vi "File_ToClass.vi"(8 "error in (no error)":errorcluster, 11 "Item Ref in":T1 format="%.0x") -> (0 "error out":errorcluster, 2 "Channels":T1[](array[typedef]) format="%.0x", 3 "File out":refnum<class "File.lvclass">)   [LabVIEW 2024, in "Embedded TDMS Logger System Explorer.lvlib"]
doc: "Creates a file class from the VeriStand System Definition File Custom Device defined by the item ref in."
uses:
  Embedded TDMS Logger System Explorer.lvlib
  <vilib>/NI VeriStand/Custom Device API/Custom Device Item Ref.ctl
  Shared/File Classes/File/File.lvclass
  Shared/File Classes/Meta Data.ctl
  <vilib>/NI VeriStand/Custom Device API/Get Item Property (String).vi
  <vilib>/NI VeriStand/Custom Device API/Get Item Property (Variant).vi
  Shared/Constants.vi
  Shared/File Classes/Group/Group.lvclass
  <vilib>/NI VeriStand/Custom Device API/Custom Device API.lvlib
  Shared/Embedded TDMS Logger Shared.lvlib
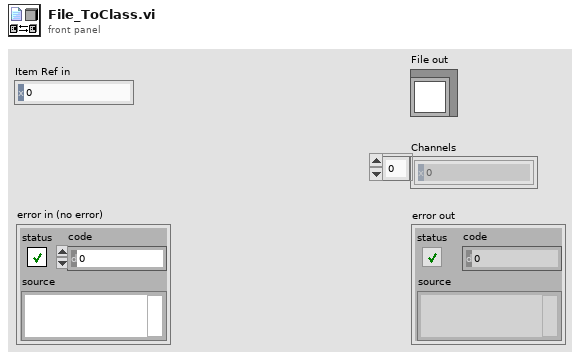
[diagram p1: front panel]
types:
  T1 = typedef "Custom Device API.lvlib/Custom Device Item Ref.ctl" = u64
  T2 = typedef "Meta Data.ctl" = cluster{"Key":string, "Value":string}
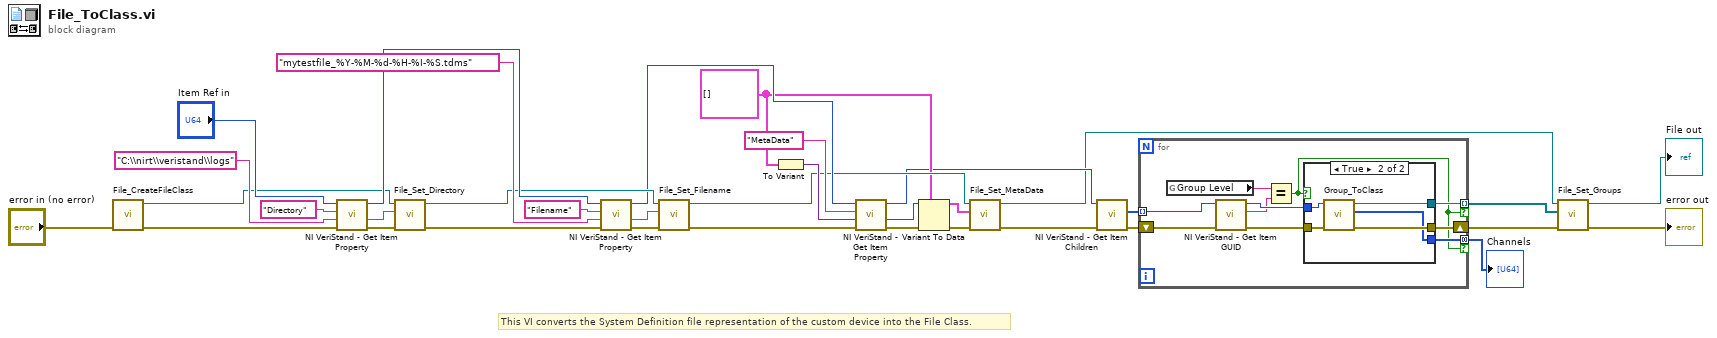
[diagram p0: block diagram]
diagram:
  w11 = T2[] []
  # "This VI converts the System Definition file representation of the custom device into the File Class."
  n1 = call "File_CreateFileClass.vi"("error in (no error)"="error in (no error)") -> ("error out"=w23:errorcluster, "File out"=w25:refnum<class "File.lvclass">)  [unwired: 9 in]
  n2 = call-poly <vilib>:"NI VeriStand - Get Item Property.vi"("error in (no error)"=w23, "Default Value"="C:\\nirt\\veristand\\logs", "Property Name"="Directory", "Item Ref in"="Item Ref in") -> ("error out"=w22:errorcluster, "Value"=w21:string, "Item Ref out"=w32:T1)  [unwired: 4 in, 1 out]
  n3 = call-dynamic "File_Set_Directory.vi"("error in (no error)"=w22, "Directory"=w21, "File in"=w25) -> ("error out"=w20:errorcluster, "File out"=w19:refnum<class "File.lvclass">)  [unwired: 7 in]
  n4 = call-poly <vilib>:"NI VeriStand - Get Item Property.vi"("error in (no error)"=w20, "Default Value"="mytestfile_%Y-%M-%d-%H-%I-%S.tdms", "Property Name"="Filename", "Item Ref in"=w32) -> ("error out"=w17:errorcluster, "Value"=w18:string, "Item Ref out"=w16:T1)  [unwired: 4 in, 1 out]
  n5 = call-dynamic "File_Set_Filename.vi"("error in (no error)"=w17, "Name"=w18, "File in"=w19) -> ("error out"=w12:errorcluster, "File out"=w13:refnum<class "File.lvclass">)  [unwired: 7 in]
  n6 = To Variant(anything=w11) -> (Variant=w29:variant)
  n7 = call-poly <vilib>:"NI VeriStand - Get Item Property.vi"("error in (no error)"=w12, "Default Value"=w29, "Property Name"="MetaData", "Item Ref in"=w16) -> ("error out"=w27:errorcluster, "Value"=w26:variant, "Item Ref out"=w10:T1)  [unwired: 4 in, 1 out]
  n8 = Variant To Data(error in=w27, type=w11, Variant=w26) -> (data=w14:T2[], error out=w15:errorcluster)
  n9 = call-dynamic "File_Set_MetaData.vi"("error in (no error)"=w15, "Meta Data"=w14, "File in"=w13) -> ("error out"=w9:errorcluster, "File out"=w2:refnum<class "File.lvclass">)  [unwired: 7 in]
  n10 = call <vilib>:"NI VeriStand - Get Item Children.vi"("error in (no error)"=w9, "Item Ref in"=w10) -> ("error out"=w8:errorcluster, "Child Refs"=w7:T1[])  [unwired: 6 in, 2 out]
  n11 = for {
    shift-right: [w41] -> w5
    shift-left: w8 -> [w45]
    tunnel: w7 -> [w44] mode=indexing
    tunnel: [w40] -> w6 mode=indexing if=w36
    tunnel: [w37] -> w1 mode=concatenating if=w36
    n12 = global read "Constants.vi" "Group Level"() -> (w39:string)
    n13 = call <vilib>:"NI VeriStand - Get Item GUID.vi"("error in (no error)"=w45, "Item Ref in"=w44) -> ("error out"=w42:errorcluster, "GUID"=w38:string, "Item Ref out"=w43:T1)  [unwired: 7 in]
    n14 = Equal?(x=w39, y=w38) -> (x = y?=w36:bool)
    n15 = case shown="True" w36 {
      tunnel: w42 -> [w46 w51]
      tunnel: w43 -> [_ w50]
      tunnel: [w46 w49] -> w41
      tunnel: [_ w48] -> w40
      tunnel: [_ w47] -> w37
      frame False {
      }
      frame True {
        n16 = call "Group_ToClass.vi"("error in (no error)"=w51, "Item Ref in"=w50) -> ("error out"=w49:errorcluster, "Channels"=w47:T1[], "Group out"=w48:refnum<class "Group.lvclass">)  [unwired: 7 in]
      }
    }
  }
  "Channels" <- w1
  n17 = call-dynamic "File_Set_Groups.vi"("error in (no error)"=w5, "Groups"=w6, "File in"=w2) -> ("error out"=→"error out":errorcluster, "File out"=→"File out":refnum<class "File.lvclass">)  [unwired: 7 in]
